vi "DestroyClone.vi"(8 "error in (no error)":errorcluster, 9 "Exit via Stop Module Req?":bool, 10 "Wait for Module to stop?":bool, 11 "ModuleAdmin":refnum<class "ModuleAdmin.lvclass">) -> (0 "error out":errorcluster, 1 "External Launch":bool, 3 "Mod Admin out":refnum<class "ModuleAdmin.lvclass">)   [LabVIEW 2014, in "AnalysisModule.lvlib"]
uses:
  AnalysisModule.lvlib
  <userlib>/NIST/ModuleAdminLib/ModuleAdmin/ModuleAdmin.lvclass
  <userlib>/NIST/ModuleAdminLib/ModuleAdmin/ModuleAdmin.lvclass/ModuleAdmin.ctl
  <userlib>/NIST/ModuleAdminLib/ModuleAdmin/Accessors/Read CloneRegRef.vi
  <userlib>/NIST/ModuleAdminLib/CloneRegistration/CloneRegistration.lvclass
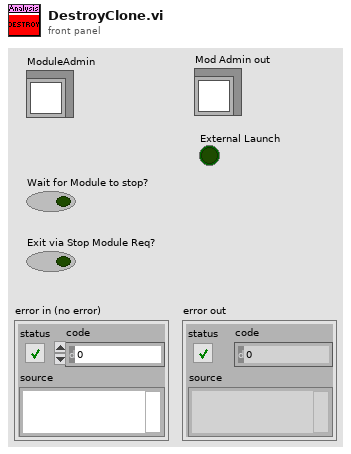
[diagram p1: front panel]
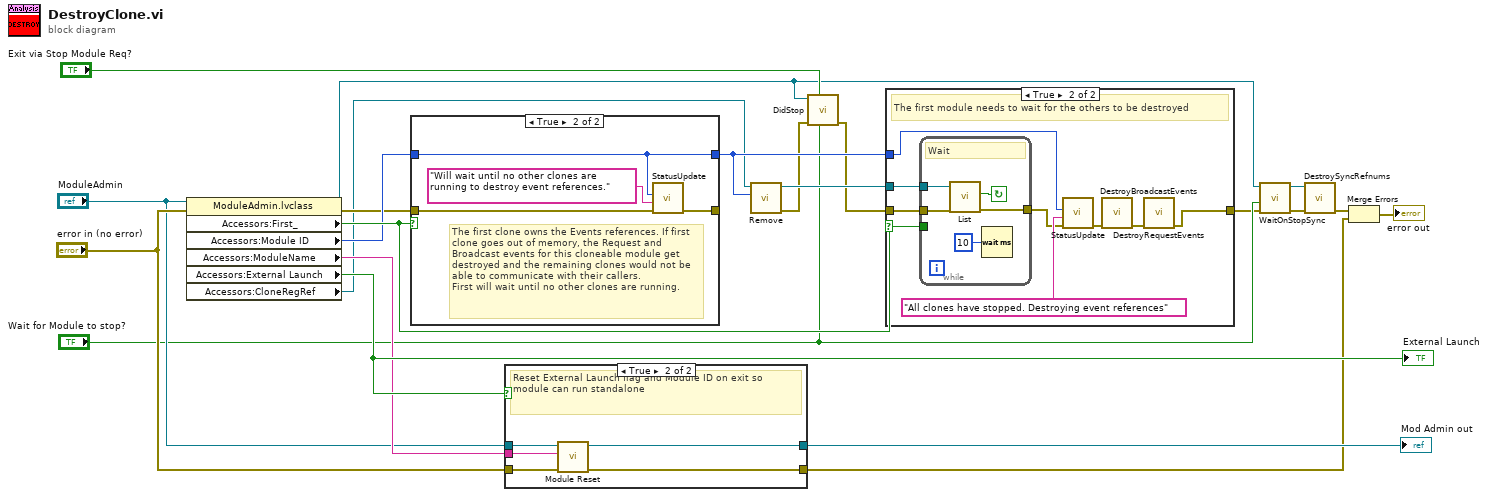
[diagram p0: block diagram]
diagram:
  n1 = property class="ModuleAdmin.lvclass"(reference="ModuleAdmin", error in="error in (no error)") -> (reference out=w1:refnum<class "ModuleAdmin.lvclass">, error out=w11:errorcluster, "Accessors:First_"=w22:bool, "Accessors:Module ID"=w14:i32, "Accessors:ModuleName"=w18:string, "Accessors:External Launch"=w20:bool, "Accessors:CloneRegRef"=w5:refnum<data-value>)
  "External Launch" <- w20
  n2 = case shown="True" w22 {
    tunnel: w11 -> [w24 w28]
    tunnel: w14 -> [w23 w25]
    tunnel: [w24 w26] -> _
    tunnel: [w23 w25] -> w21
    frame False {
    }
    frame True {
      # "The first clone owns the Events references. If first clone goes out of memory, the Request and Broadcast events for this cloneable module get destroyed and the remaining clones would not be able to communicate with their callers.\nFirst will wait until no other clones are running."
      n3 = call "StatusUpdate.vi"("error in (no error)"=w28, "Status"="Will wait until no other clones are running to destroy event references." ("format string"), "ModuleID"=w25) -> ("error out"=w26:errorcluster)  [unwired: 8 in]
    }
  }
  n4 = case shown="True" w20 {
    tunnel: "error in (no error)" -> [w29 w35]
    tunnel: w18 -> [_ w34]
    tunnel: "ModuleAdmin" -> [w30 w33]
    tunnel: [w30 w32] -> w17
    tunnel: [w29 w31] -> w15
    frame False {
    }
    frame True {
      # "Reset External Launch flag and Module ID on exit so module can run standalone"
      n5 = call <userlib>:"Module Reset.vi"("error in (no error)"=w35, "ModuleName"=w34, "Mod Admin in"=w33) -> ("error out"=w31:errorcluster, "Mod Admin out"=w32:refnum<class "ModuleAdmin.lvclass">)  [unwired: 7 in]
    }
  }
  "Mod Admin out" <- w17
  n6 = call <userlib>:"Remove.vi"("Module ID"=w21, "CloneRegRef"=w5) -> ("error out"=w10:errorcluster, "CloneRegRef"=w13:refnum<data-value>)  [unwired: 7 in, 1 out]
  n7 = call "DidStop.vi"("Wait for Module to stop?"="Wait for Module to stop?", "Exit via Stop Module Req?"="Exit via Stop Module Req?", "error in (no error)"=w10, "ModuleAdmin"=w1) -> ("error out"=w9:errorcluster)  [unwired: 7 in]
  n8 = case shown="True" w22 {
    selector: w22 -> [_ w44]
    tunnel: w9 -> [w36 w45]
    tunnel: w21 -> [_ w39]
    tunnel: [w36 w37] -> w4
    tunnel: w13 -> [_ w38]
    frame False {
    }
    frame True {
      # "The first module needs to wait for the others to be destroyed"
      n9 = while {
        tunnel: w45 -> [w50]
        tunnel: w44 -> [_]
        tunnel: [w49] -> w42
        tunnel: w38 -> [w46]
        stop <- w48 continue-if-true
        # "Wait"
        n10 = call <userlib>:"List.vi"("error in (no error)"=w50, "CloneRegRef"=w46) -> ("error out"=w49:errorcluster, "Found?"=w48:bool)  [unwired: 4 in, 4 out]
        n11 = Wait (ms)(milliseconds to wait=u32 10) -> ()  [unwired: 1 out]
      }
      n12 = call "StatusUpdate.vi"("error in (no error)"=w42, "Status"="All clones have stopped. Destroying event references", "ModuleID"=w39) -> ("error out"=w41:errorcluster)  [unwired: 8 in]
      n13 = call "DestroyBroadcastEvents.vi"("error in (no error)"=w41) -> ("error out"=w40:errorcluster)  [unwired: 10 in]
      n14 = call "DestroyRequestEvents.vi"("error in (no error)"=w40) -> ("error out"=w37:errorcluster)  [unwired: 10 in]
    }
  }
  n15 = call <userlib>:"WaitOnStopSync.vi"("error in (no error)"=w4, "WaitForModuleToStop?"="Wait for Module to stop?", "ModuleAdmin"=w1) -> ("error out"=w3:errorcluster, "ModuleAdmin"=w8:refnum<class "ModuleAdmin.lvclass">)  [unwired: 7 in]
  n16 = call <userlib>:"DestroySyncRefnums.vi"("error in (no error)"=w3, "ModuleAdmin"=w8) -> ("error out"=w2:errorcluster)  [unwired: 9 in]
  n17 = Merge Errors(w2, w15) -> (→"error out":errorcluster)
